vi "Write Name.vi"(8 "error in (no error)":errorcluster, 10 "Name":string, 11 "Loop in":refnum<class "Loop.lvclass">) -> (0 "error out":errorcluster, 3 "Loop out":refnum<class "Loop.lvclass">)   [LabVIEW 2024, in "Ramses Sequencer.lvlib" / "Loop.lvclass"]
uses:
  Loop.lvclass
  Loop.lvclass/Loop.ctl
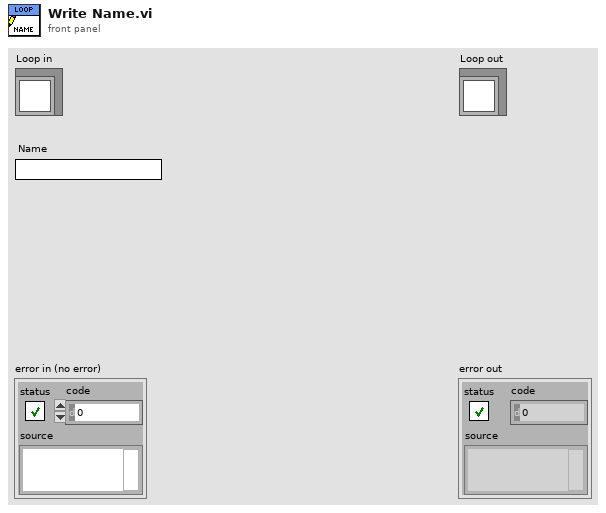
[diagram p1: front panel]
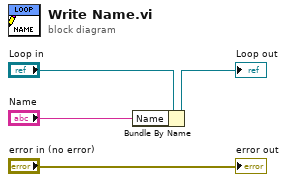
[diagram p0: block diagram]
diagram:
  n1 = Bundle By Name(cluster="Loop in", "Name"="Name") -> (→"Loop out":refnum<class "Loop.lvclass">)
  "error out" <- "error in (no error)"
